vi "Get Conn Status Chan Path.vi"(3 "Link":T1) -> (0 "Empty Link?":bool, 1 "Conn Status Chan":string)   [LabVIEW 2011]
uses:
  Controls/ECUMC Item.ctl
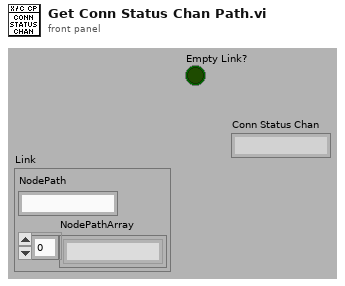
[diagram p1: front panel]
types:
  T1 = typedef "ECUMC Item.ctl" = cluster{"NodePath":string, "NodePathArray":string[]}
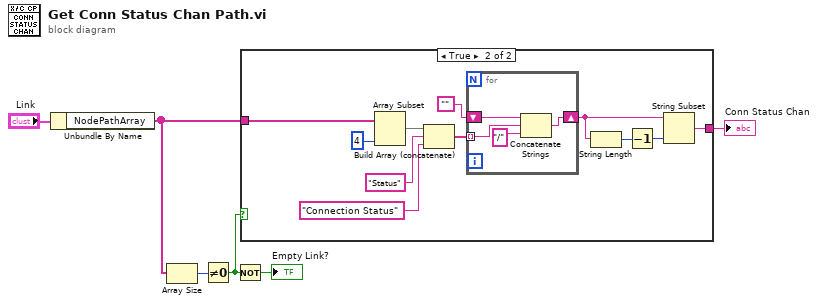
[diagram p0: block diagram]
diagram:
  n1 = Unbundle By Name("Link") -> ("NodePathArray"=w4:string[])
  n2 = Array Size(array=w4) -> (size(s)=w3:i32)
  n3 = Not Equal To 0?(x=w3) -> (x != 0?=w2:bool)
  n4 = Not(x=w2) -> (.not. x?=→"Empty Link?":bool)
  n5 = case shown="True" w2 {
    tunnel: [_ w17] -> w6
    tunnel: w4 -> [_ w7]
    frame False {
    }
    frame True {
      n6 = Array Subset(array=w7, length=4) -> (w15:string[])  [unwired: 1 in]
      n7 = Build Array (concatenate)(w15, "Status" ("input 3"), "Connection Status" ("input 4")) -> (w12:string[])
      n8 = for {
        tunnel: w12 -> [w20] mode=indexing
        shift-right: [w18] -> w10
        shift-left: "" -> [w21]
        n9 = Concatenate Strings(w21, w20, "/" ("string")) -> (w18:string)
      }
      n10 = String Length(string=w10) -> (length=w9:i32)
      n11 = Decrement(x=w9) -> (x-1=w8:i32)
      n12 = String Subset(string=w10, length (rest)=w8) -> (substring=w17:string)  [unwired: 1 in]
    }
  }
  "Conn Status Chan" <- w6
